vi "Set Topology Property.vi"(8 "error in":errorcluster, 10 "topology":string, 11 "slsc switch custom device in":T1 format="%.0x") -> (0 "error out":errorcluster, 3 "slsc switch custom device out":T1 format="%.0x")   [LabVIEW 2020, in "SLSC Switch Scripting.lvlib"]
uses:
  SLSC Switch Scripting.lvlib
  <vilib>/NI VeriStand/Custom Device API/Custom Device Item Ref.ctl
  SLSC Scripting Constants.vi
  <vilib>/NI VeriStand/Custom Device API/Set Item Property (String).vi
  <vilib>/NI VeriStand/Custom Device API/Custom Device API.lvlib
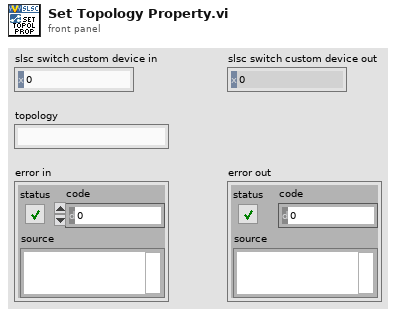
[diagram p1: front panel]
types:
  T1 = typedef "Custom Device API.lvlib/Custom Device Item Ref.ctl" = u64
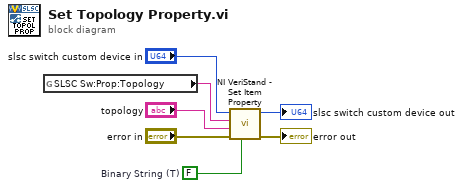
[diagram p0: block diagram]
diagram:
  w4 = FALSE  # Binary String (T)
  n1 = global read "SLSC Scripting Constants.vi" "SLSC Sw:Prop:Topology"() -> (w3:string)
  n2 = call-poly <vilib>:"NI VeriStand - Set Item Property.vi"("Binary String (T)"=w4, "error in (no error)"="error in", "Value"="topology", "Property Name"=w3, "Item Ref in"="slsc switch custom device in") -> ("error out"=→"error out":errorcluster, "Item Ref out"=→"slsc switch custom device out":T1)  [unwired: 4 in, 1 out]
